vi "CloseListener.vi"(0 "TCP Socket in":refnum<class "Socket Communication.lvclass">, 5 "error in (no error)":errorcluster) -> (14 "TCP Socket out":refnum<class "Socket Communication.lvclass">, 19 "error out":errorcluster)   [LabVIEW 2016, in "Socket Communication.lvclass"]
uses:
  Socket Communication.lvclass
  Socket Communication.lvclass/Socket Communication.ctl
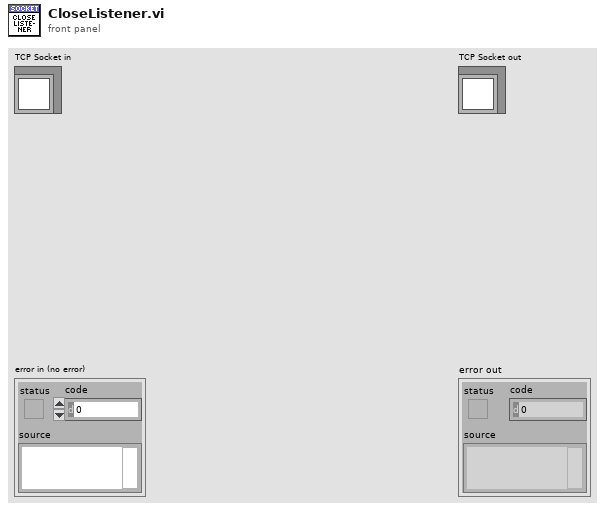
[diagram p1: front panel]
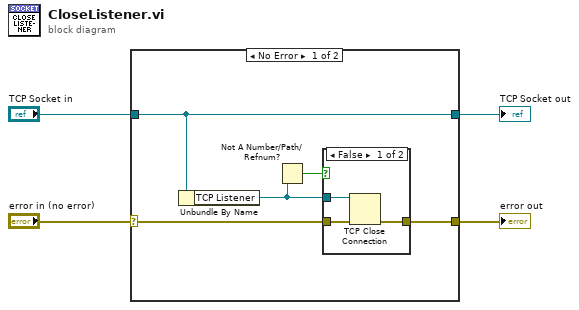
[diagram p0: block diagram]
diagram:
  n1 = case shown="No Error" "error in (no error)" {
    selector: "error in (no error)" -> [w8 w15]
    tunnel: [w7 w15] -> w3
    tunnel: [w9 w14] -> w1
    tunnel: "TCP Socket in" -> [w9 w14]
    frame No Error {
      n2 = Unbundle By Name(w9) -> ("TCP Listener"=w6:refnum<k5>)
      n3 = Not A Number/Path/Refnum?(number/path/refnum=w6) -> (NaN/Path/Refnum?=w5:bool)
      n4 = case shown="False" w5 {
        tunnel: w8 -> [w12 w13]
        tunnel: [w11 w13] -> w7
        tunnel: w6 -> [w10 _]
        frame False {
          n5 = TCP Close Connection(connection ID=w10, error in (no error)=w12) -> (error out=w11:errorcluster)  [unwired: 1 in, 1 out]
        }
        frame True {
        }
      }
    }
    frame Error {
    }
  }
  "error out" <- w3
  "TCP Socket out" <- w1
